vi "Set Number of Cameras.vi"(8 "error in (no error)":errorcluster, 10 "Cameras":i32, 11 "Application in":refnum<class "Application.lvclass">) -> (0 "error out":errorcluster, 3 "Application out":refnum<class "Application.lvclass">)   [LabVIEW 2015, in "Application.lvlib" / "Application.lvclass"]
uses:
  Application.lvclass
  Application.lvclass/Application.ctl
  User Interface/Main Window Messages/Set Number of Cameras Msg/Set Number of Cameras Msg.lvclass/Set Number of Cameras Msg.ctl
  <vilib>/ActorFramework/Message Enqueuer/Message Enqueuer.lvclass/Message Enqueuer.ctl
  <vilib>/ActorFramework/Message Enqueuer/Enqueue.vi
  <vilib>/ActorFramework/Message Priority Queue/Priority Enqueue.vi
  User Interface/Main Window Messages/Set Number of Cameras Msg/Set Number of Cameras Msg.lvclass
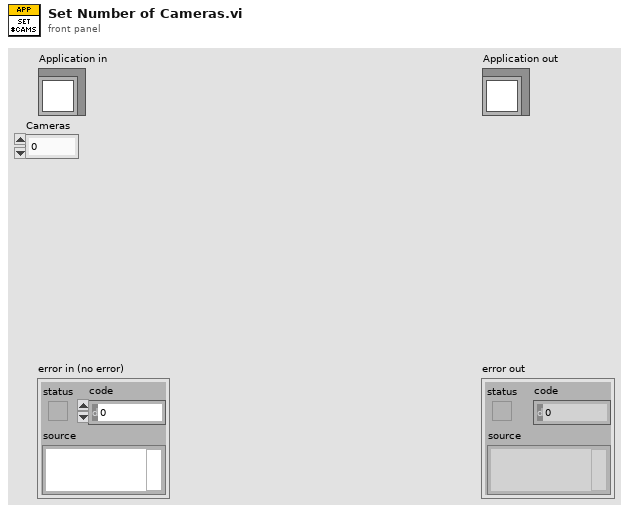
[diagram p1: front panel]
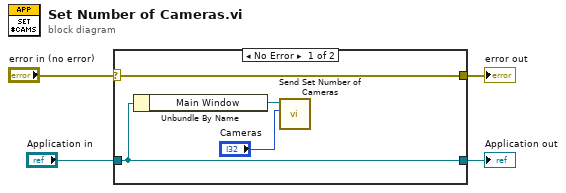
[diagram p0: block diagram]
diagram:
  n1 = case shown="No Error" "error in (no error)" {
    selector: "error in (no error)" -> [w8 w10]
    tunnel: [w8 w10] -> w3
    tunnel: [w7 w9] -> w1
    tunnel: "Application in" -> [w7 w9]
    frame No Error {
      n2 = Unbundle By Name(w7) -> ("Main Window"=w6:refnum<class "Message Enqueuer.lvclass">)
      n3 = call "Send Set Number of Cameras.vi"("Cameras"="Cameras", "Message Enqueuer"=w6) -> ()  [unwired: 8 in, 2 out]
    }
    frame Error {
    }
  }
  "error out" <- w3
  "Application out" <- w1
